vi "3458A Build Unique Identifiers.vi"(8 "error in":errorcluster, 10 "dmm(s) idn strings in":string[](array[string]), 11 "digitizer session in":T1 {"channels"."Range [Vpk]" min=0.0}) -> (0 "error out":errorcluster, 1 "display strings":string[](array[string]), 2 "identifier strings":string[](array[string]), 3 "digitizer session out":T1 {"channels"."Range [Vpk]" min=0.0})   [LabVIEW 2013, in "3458A Virtual Digitizer.lvlib"]
doc: "3458A digitize lib: This VI tries to build unique identifiers of the 3458A units. Depending on the mode of identification it will try to build the idn from CALSTR command response or just sequentially numbers the channels. When s.n. extracted from CALSTR? are not unique it will generate error."
uses:
  3458A Virtual Digitizer.lvlib
  3458A Digitizer Session.ctl
  3458A Virtual Channel Config.ctl
  Counter/Counter Session.ctl
  Counter/Counter Type.ctl
  AWG/AWG Session.ctl
  AWG/AWG Type.ctl
  3458A Sync Mode.ctl
  3458A Idn Mode.ctl
  3458A Digitizing Low Levels/Configure/Sampling Mode.ctl
  3458A Digitizing Process Options.ctl
  3458A Data Packet.ctl
  3458A Aux Record Data.ctl
  3458A Digitizing Low Levels/Configure/Level Setup.ctl
  3458A Digitizing Low Levels/Configure/First Sample Trigger.ctl
  <vilib>/Utility/error.llb/Error Cluster From Error Code.vi
  <vilib>/ErrorRing/Error Ring.xnode
  3458A Digitizing Low Levels/3458A Digitizing Low Levels.lvlib
  Counter/Counter.lvlib
  AWG/AWG.lvlib
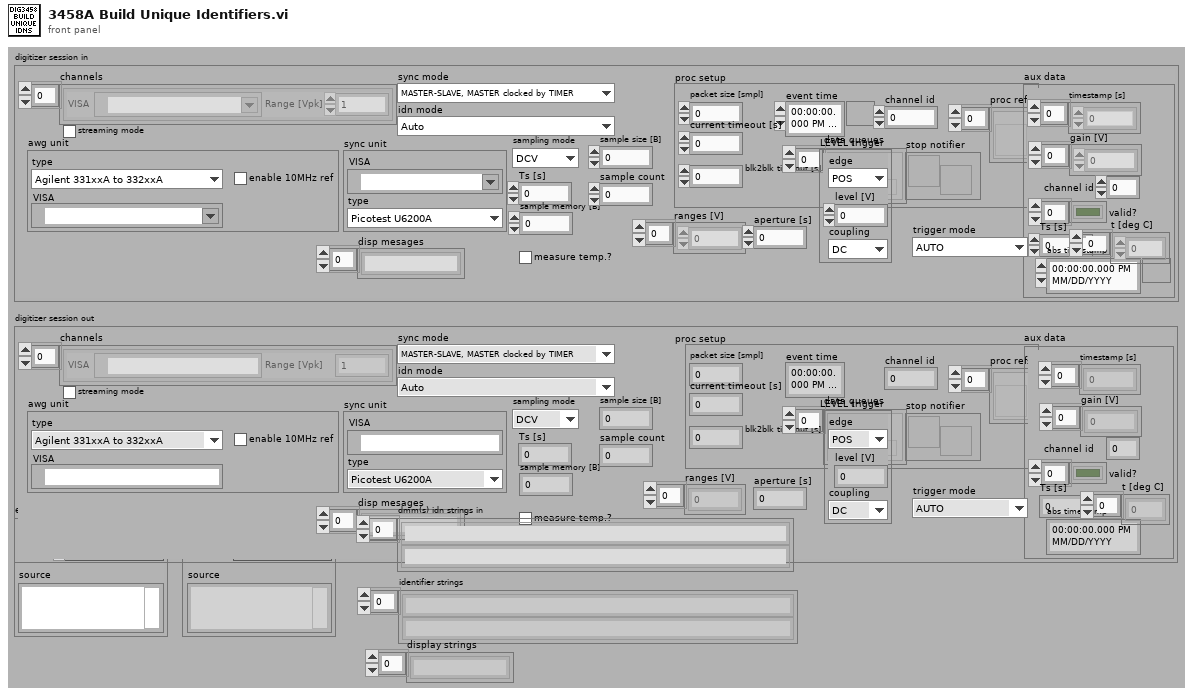
[diagram p1: front panel]
types:
  T1 = typedef "3458A Virtual Digitizer.lvlib/3458A Digitizer Session.ctl" = cluster{"channels":T2[], "sync unit":T3, "awg unit":T5, "sync mode":T7, "streaming mode":bool, "idn mode":T8, "sampling mode":T9, "Ts [s]":dbl, "sample memory [B]":i32, "proc setup":T10, "sample size [B]":i32, "sample count":i32, "aux data":T11, "ranges [V]":dbl[], "aperture [s]":dbl, "LEVEL trigger":T12, "trigger mode":T13, "measure temp.?":bool, "disp mesages":string[]}
  T2 = typedef "3458A Virtual Digitizer.lvlib/3458A Virtual Channel Config.ctl" = cluster{"VISA":refnum<visa-resource-name>, "Range [Vpk]":dbl}
  T3 = typedef "Counter.lvlib/Counter Session.ctl" = cluster{"VISA":refnum<visa-resource-name>, "type":T4}
  T4 = typedef "Counter.lvlib/Counter Type.ctl" = enum16{"Picotest U6200A", "dummy"}
  T5 = typedef "AWG.lvlib/AWG Session.ctl" = cluster{"type":T6, "VISA":refnum<visa-resource-name>, "enable 10MHz ref":bool}
  T6 = typedef "AWG.lvlib/AWG Type.ctl" = enum16{"Agilent 331xxA to 332xxA", "Agilent 335xxA to 336xxA", "dummy"}
  T7 = typedef "3458A Virtual Digitizer.lvlib/3458A Sync Mode.ctl" = enum16{"MASTER-SLAVE, MASTER clocked by TIMER", "MASTER-SLAVE, MASTER clocked by AWG", "ALL clocked by AWG", "MASTER-SLAVE, ALL clocked by TIMER", "ALL clocked by AWG with DFLL"}
  T8 = typedef "3458A Virtual Digitizer.lvlib/3458A Idn Mode.ctl" = enum16{"Auto", "Sequential (chn A, chn B, ...)", "From calibration string"}
  T9 = typedef "3458A Virtual Digitizer.lvlib/3458A Digitizing Low Levels.lvlib/Sampling Mode.ctl" = enum16{"DCV", "DSDC", "DSAC"}
  T10 = typedef "3458A Virtual Digitizer.lvlib/3458A Digitizing Process Options.ctl" = cluster{"channel id":i32, "packet size [smpl]":i32, "current timeout [s]":dbl, "blk2blk timeout [s]":dbl, "event time":timestamp, "stop notifier":refnum<notifier>, "data queues":refnum<queue>[], "proc refs":refnum<vi>[]}
  T11 = typedef "3458A Virtual Digitizer.lvlib/3458A Aux Record Data.ctl" = cluster{"channel id":i32, "valid?":bool[], "gain [V]":dbl[], "timestamp [s]":dbl[], "Ts [s]":dbl, "abs timestamp":timestamp, "t [deg C]":dbl[]}
  T12 = typedef "3458A Virtual Digitizer.lvlib/3458A Digitizing Low Levels.lvlib/Level Setup.ctl" = cluster{"edge":enum16{"POS", "NEG"}, "level [V]":dbl, "coupling":enum16{"DC", "AC"}}
  T13 = typedef "3458A Virtual Digitizer.lvlib/3458A Digitizing Low Levels.lvlib/First Sample Trigger.ctl" = enum16{"AUTO", "EXT", "SYN", "SGL", "HOLD", "LEVEL"}
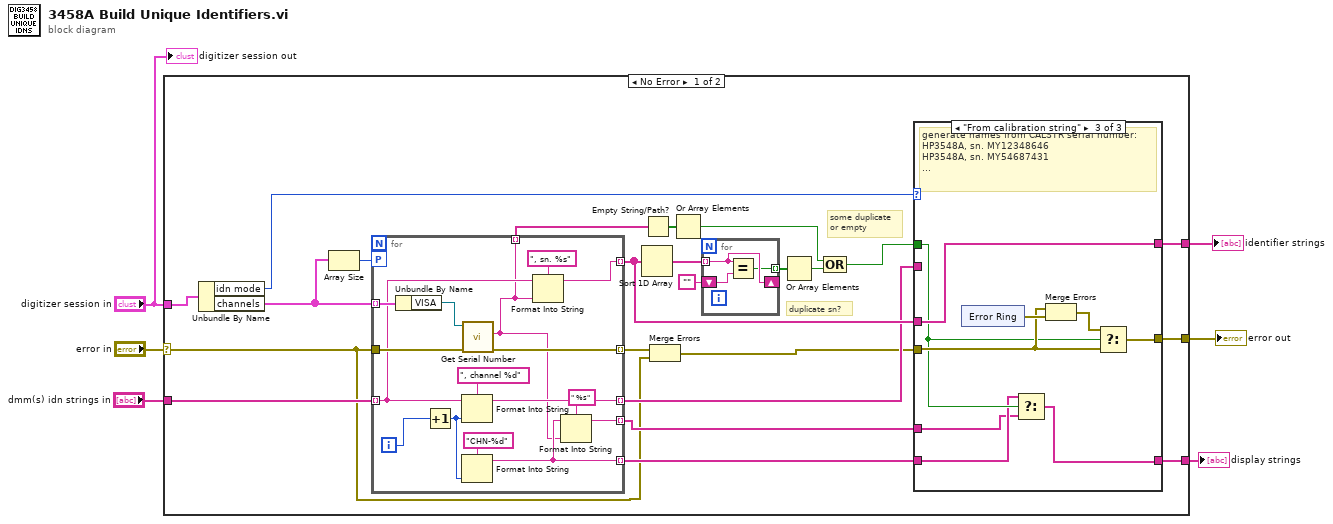
[diagram p0: block diagram]
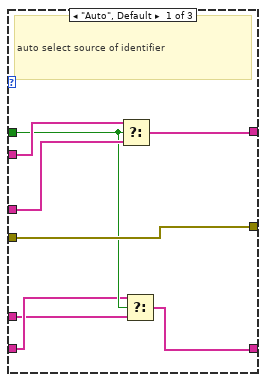
[diagram p2: hidden frame]
diagram:
  n1 = case shown="No Error" "error in" {
    selector: "error in" -> [w7 w75]
    tunnel: "digitizer session in" -> [w29 _]
    tunnel: "dmm(s) idn strings in" -> [w16 w74]
    tunnel: [w13 w75] -> w5
    tunnel: [w12 w74] -> w4
    tunnel: [w9 _] -> w1
    frame No Error {
      # "some duplicate\nor empty"
      # "duplicate sn?"
      n2 = Unbundle By Name(w29) -> ("idn mode"=w19:T8, "channels"=w28:T2[])
      n3 = Array Size(array=w28) -> (size(s)=w27:i32)
      n4 = for {
        tunnel: w7 -> [w73]
        tunnel: w28 -> [w72] mode=indexing
        workers-P: w27 -> [_]
        tunnel: [w70] -> w26 mode=indexing
        tunnel: [w65] -> w18 mode=indexing
        tunnel: [w67] -> w17 mode=indexing
        tunnel: w16 -> [w64] mode=indexing
        tunnel: [w59] -> w11 mode=indexing
        tunnel: [w60] -> w10 mode=indexing
        tunnel: [w58] -> w8 mode=indexing
        i -> [w68]
        n5 = Unbundle By Name(w72) -> ("VISA"=w71:refnum<visa-resource-name>)
        n6 = Increment(x=w68) -> (x+1=w62:i32)
        n7 = Format Into String(format string=", channel %d", initial string=w64, w62) -> (resulting string=w67:string)  [unwired: 1 in, 1 out]
        n8 = Format Into String(format string="CHN-%d", w62) -> (resulting string=w60:string)  [unwired: 2 in, 1 out]
        n9 = call "Get Serial Number.vi"("error in"=w73, "VISA resource in"=w71) -> ("error out"=w70:errorcluster, "serial number"=w59:string)  [unwired: 5 in, 3 out]
        n10 = Format Into String(format string=", sn. %s", initial string=w64, w59) -> (resulting string=w65:string)  [unwired: 1 in, 1 out]
        n11 = Format Into String(format string=" %s", initial string=w60, w59) -> (resulting string=w58:string)  [unwired: 1 in, 1 out]
      }
      n12 = Sort 1D Array(array=w18) -> (sorted array=w25:string[])
      n13 = Empty String/Path?(string/path=w11) -> (empty?=w21:bool[])
      n14 = Merge Errors(w26, w7) -> (w14:errorcluster)
      n15 = Or Array Elements(Boolean array=w21) -> (logical OR=w20:bool)
      n16 = for {
        tunnel: w25 -> [w56] mode=indexing
        shift-right: [w56] -> _
        shift-left: "" -> [w57]
        tunnel: [w55] -> w23 mode=indexing
        n17 = Equal?(x=w56, y=w57) -> (x = y?=w55:bool)
      }
      n18 = Or Array Elements(Boolean array=w23) -> (logical OR=w22:bool)
      n19 = Compound Arithmetic op=OR(w20, w22) -> (w15:bool)
      n20 = case shown="\"From calibration string\"" w19 {
        tunnel: w18 -> [w35 _ w49]
        tunnel: w17 -> [w36 w40 _]
        tunnel: [w37 w40 w49] -> w12
        tunnel: w15 -> [w33 _ w44]
        tunnel: w14 -> [w34 w39 w46]
        tunnel: [w34 w39 w45] -> w13
        tunnel: w10 -> [w32 w38 w43]
        tunnel: [w30 w38 w41] -> w9
        tunnel: w8 -> [w31 _ w42]
        frame "Auto", Default {
          # "auto select source of identifier"
          n21 = Select(t=w36, s=w33, f=w35) -> (s? t:f=w37:string[])
          n22 = Select(t=w32, s=w33, f=w31) -> (s? t:f=w30:string[])
        }
        frame "Sequential (chn A, chn B, ...)" {
          # "generate sequential names:\nHP3548A, channel 1\nHP3548A, channel 2\n..."
        }
        frame "From calibration string" {
          # "generate names from CALSTR serial number:\nHP3548A, sn. MY12348646\nHP3548A, sn. MY54687431\n..."
          n23 = xnode "Error Ring"() -> ("error out"=w48:errorcluster)
          n24 = Select(t=w43, s=w44, f=w42) -> (s? t:f=w41:string[])
          n25 = Merge Errors(w46, w48) -> (w47:errorcluster)
          n26 = Select(t=w47, s=w44, f=w46) -> (s? t:f=w45:errorcluster)
        }
      }
    }
    frame Error {
    }
  }
  "error out" <- w5
  "identifier strings" <- w4
  "display strings" <- w1
  "digitizer session out" <- "digitizer session in"
